vi "XY Graph Set Tool Panels Visibility.vi"(8 "error in (no error)":errorcluster, 10 "Graph Tool Panels Visibility":T1, 11 "XYGraph in":T2) -> (0 "error out":errorcluster, 3 "XYGraph out":T2)   [LabVIEW 2021, in "XY Graph Add-Ons.lvlib"]
uses:
  XY Graph Add-Ons.lvlib
  XY Graph Refnum.ctl
  XY Graph Tool Panels Visibility.ctl
  XY Graph Property Tag List.ctl
  <vilib>/UserTags/UserTags.lvlib
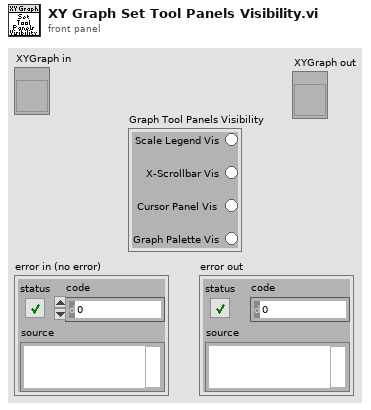
[diagram p1: front panel]
types:
  T1 = typedef "XY Graph Add-Ons.lvlib/XY Graph Tool Panels Visibility.ctl" = cluster{"Scale Legend Vis":bool, "X-Scrollbar Vis":bool, "Cursor Panel Vis":bool, "Graph Palette Vis":bool}
  T2 = typedef "XY Graph Add-Ons.lvlib/XY Graph Refnum.ctl" = refnum<vi>
  T3 = typedef "XY Graph Add-Ons.lvlib/XY Graph Property Tag List.ctl" = enum16{"Max Legend Size", "Preserved Plots", "XScales.GridColors", "YScales.GridColors", "TipStrip String", "TipStrip Visible", "Tool Panels Visibility", "Plots Metadata"}
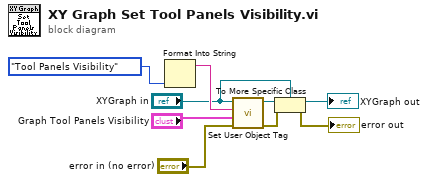
[diagram p0: block diagram]
diagram:
  n1 = Format Into String(XY_Graph_Property_Tag_List."Tool Panels Visibility" ("XY Graph Property Tag")) -> (resulting string=w9:string)  [unwired: 3 in, 1 out]
  n2 = call <vilib>:"Set User Object Tag.vi"("error in (no error)"="error in (no error)", "Value"="Graph Tool Panels Visibility", "Tag Name"=w9, "Generic Refnum"="XYGraph in") -> ("error out"=w3:errorcluster, "dup Generic Refnum"=w6:refnum<vi>)  [unwired: 5 in, 1 out]
  n3 = To More Specific Class(target class="XYGraph in", reference=w6, error in=w3) -> (specific class reference=→"XYGraph out":T2, error out=→"error out":errorcluster)
